vi "適應性控制_輸入權重係數+數位積分_隔振V3(實際控制).vi"() -> ()   [LabVIEW 2010]
uses:
  <vilib>/DAQmx/read.llb/DAQmx Read (Analog DBL 1Chan 1Samp).vi
  <vilib>/DAQmx/write.llb/DAQmx Write (Analog DBL 1Chan 1Samp).vi
  <vilib>/DAQmx/create/channels.llb/DAQmx Create Channel (AI-Voltage-Basic).vi
  <vilib>/DAQmx/configure/timing.llb/DAQmx Timing (Sample Clock).vi
  <vilib>/DAQmx/create/channels.llb/DAQmx Create Channel (AO-Voltage-Basic).vi
  <vilib>/daqmx/miscellaneous.llb/DAQmx Fill In Error Info.vi
  <vilib>/measure/maspectr.llb/FFT Spectrum (Mag-Phase) for 1 Chan.vi
  <vilib>/measure/NI_MAPro.lvlib
panel:
  out "當下頻率":dbl
  out "max value":dbl
  out "phase":cluster{"f0":dbl, "df":dbl, "phase":dbl[]} {"phase" format="%.2p"; "f0" format="%0.2p"; "df" format="%0.2p"}
  in  "averaging parameters 2":T1={"averaging mode"=enum."No averaging", "weighting mode"=enum."Exponential", "number of averages"=10} {"number of averages" min=1}
  out "Waveform Graph 2":cluster{"f0":dbl, "df":dbl, "magnitude":dbl[]}(graph)
  in  "資料數":i32
  in  "權重":dbl[][](array[numeric])=array3077x82[252314 elements]
  in  "輸出DC濾除":dbl
  out "當前權重":dbl[](array[numeric])
  in  "相位":dbl
  in  "I增益":dbl
  in  "DAQ input":tag
  in  "DAQ output":tag
  in  "平均數":i32=1
  in  "ÂoDC«á©ñ¤j":dbl=1.0
  in  "Kp":dbl
  out "當下誤差":dbl=0.1 format="%#_13g"
  out "模擬輸入x(t)":dbl[][](graph)
  out "理想與FIR輸出":dbl[][](graph)
  out "message":string=" INSTRUCTIONS:\r\rNormal Use:  When using subVIs that incorporate the error in/error out (or error I/O) structure, place this handler where you want to inform the user of an error, typically at the end of the I/O data path, as the last action of the program.  If the error in error? is ERROR, the handler creates a message describing the error and its source.  If the type of dialog = 1 (default), the message is displayed to the user, who can only acknowedge it.  If the type = 2, the user can acknowledge the message or abort execution; aborting a program with active I/O is not recommended.  If the type = 0, no message is displayed; this is used to process the error programmatically, and the error out cluster elements are wired to individual terminals for that reason.  \r\rOther Use:\n\r\nlocal testing.  To test the error code of a subVI or function that does not have the error I/O structure, you can wire its error code and a source string to the local error code and error source inputs.  If error in error? indicates no error and error code is not equal to 0, the local code and source are substituted for the error in values, and error? is set TRUE (ERROR)."
  out "誤差":dbl(graph)
  out "while平均運行時間":dbl
  out "收斂time":dbl
  out "各頻率誤差已達標準":bool
  in  "各頻率誤差低於多少亮燈":dbl=0.1 format="%#_13g"
  in  "order":i32=80
  in  "取樣頻率":dbl=1000.0 min=1.0 max=1000.0 step=1.0
  in  "stop":bool
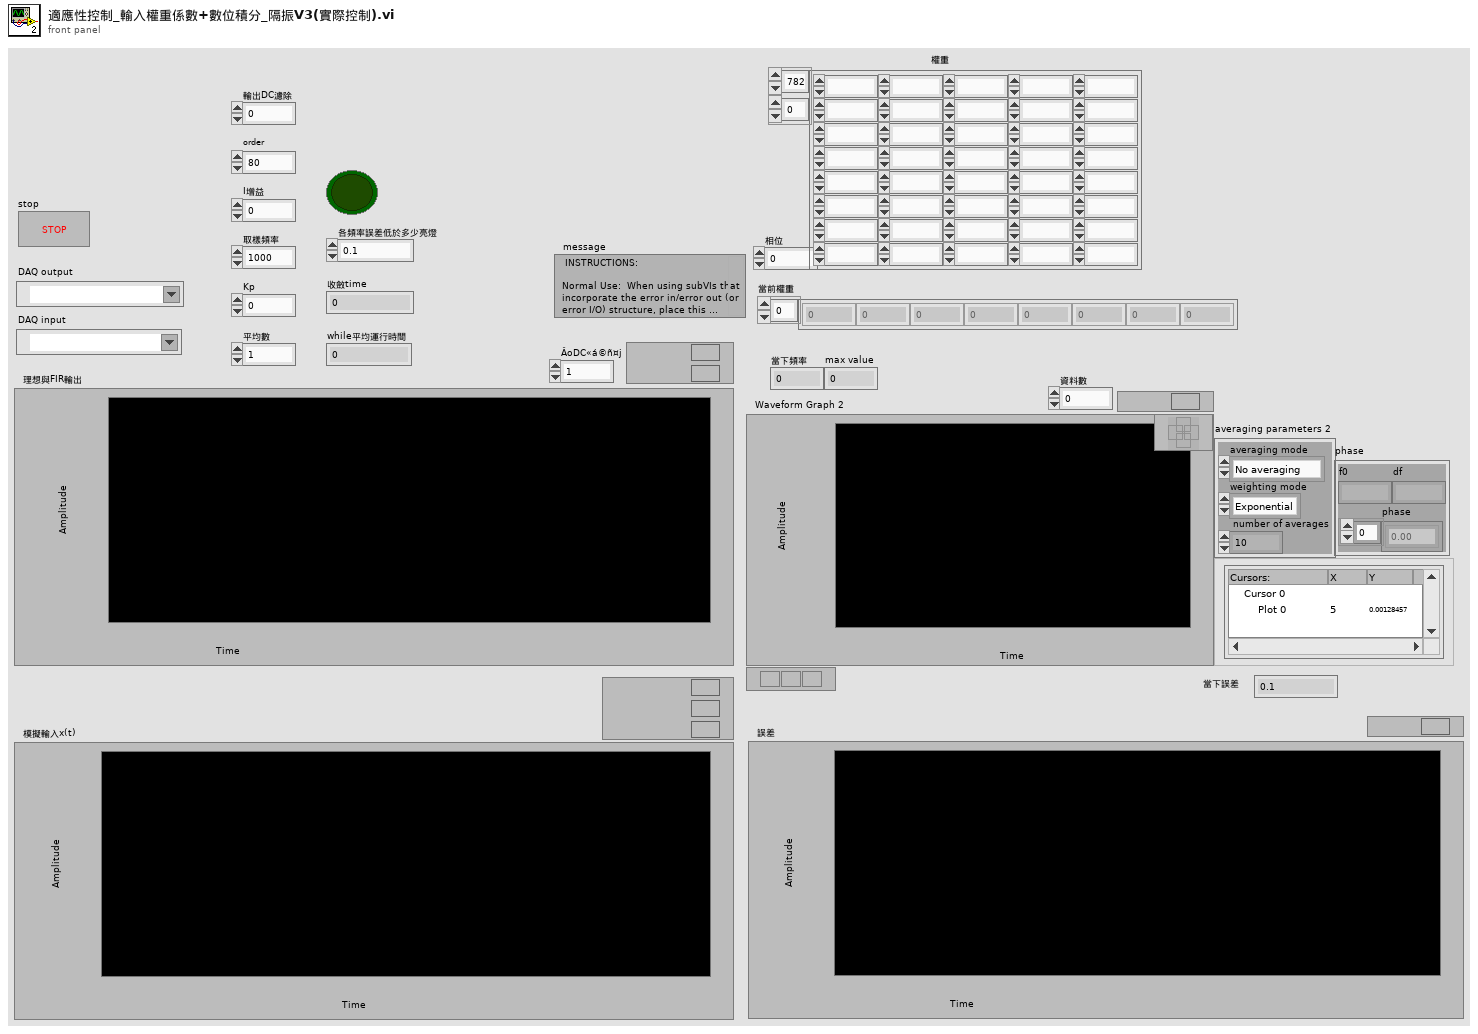
[diagram p1: front panel]
types:
  T1 = cluster{"averaging mode":enum16{"No averaging", "Vector averaging", "RMS averaging", "Peak hold"}, "weighting mode":enum16{"Linear", "Exponential"}, "number of averages":u32}
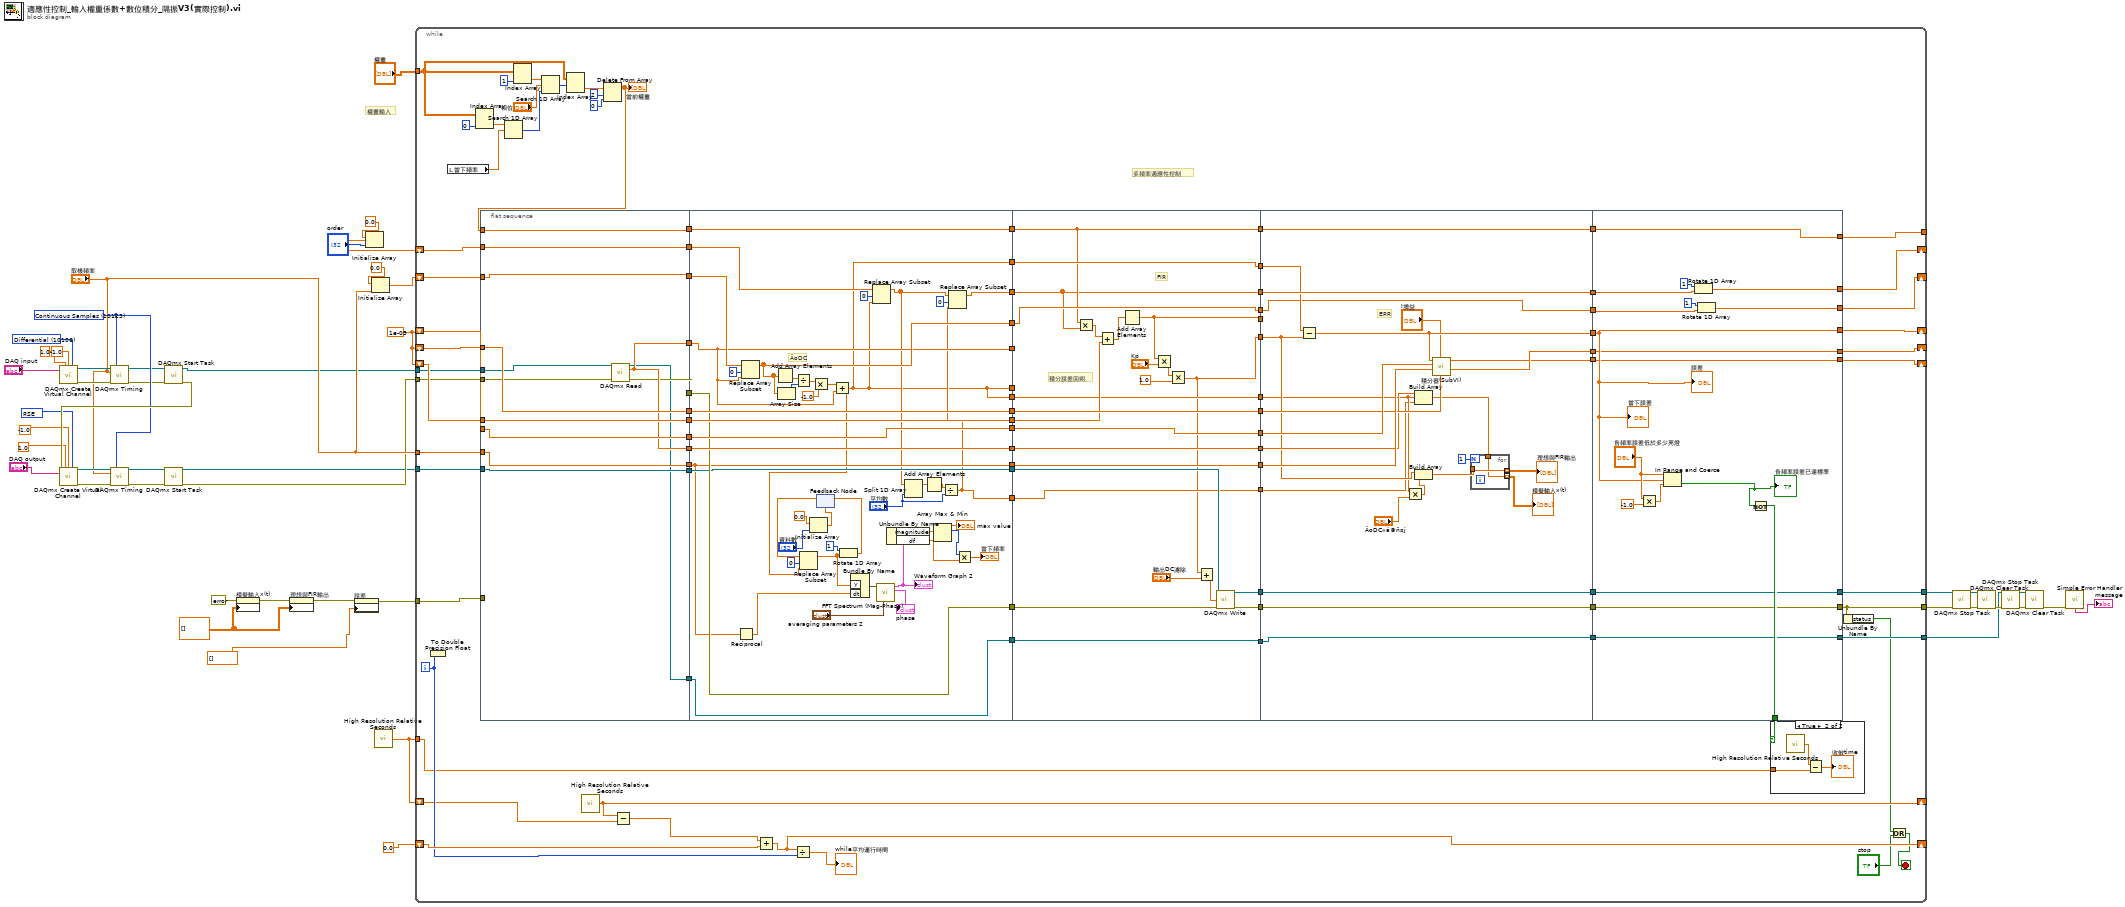
[diagram p0: block diagram]
diagram:
  w29 = 10123 items=["Finite Samples"=10178, "Continuous Samples"=10123, "Hardware Timed Single Point"=12522] ("sample mode")
  w26 = 10083 items=["Default"=-1, "RSE"=10083, "Differential"=10106, "Pseudodifferential"=12529] ("output terminal configuration")
  w25 = 10106 items=["default"=-1, "RSE"=10083, "NRSE"=10078, "Differential"=10106, "Pseudodifferential"=12529] ("input terminal configuration")
  w37 = 1e-05 ("x")
  w33 = dbl[][] [] ("History Data")
  # "權重輸入"
  n1 = call-poly <vilib>:"DAQmx Create Virtual Channel.vi"("maximum value"=1.0, "minimum value"=-1.0, "input terminal configuration"=w25, "physical channels"="DAQ input") -> ("task out"=w17:refnum<k21>, "error out"=w20:errorcluster)  [unwired: 10 in]
  n2 = call-poly <vilib>:"DAQmx Timing.vi"("task/channels in"=w17, "sample mode"=w29, "rate"="取樣頻率", "error in"=w20) -> ("task out"=w18:refnum<k21>, "error out"=w19:errorcluster)  [unwired: 10 in]
  n3 = call <vilib>:"DAQmx Start Task.vi"("task/channels in"=w18, "error in"=w19) -> ("task out"=w15:refnum<k21>, "error out"=w32:errorcluster)  [unwired: 12 in]
  n4 = call-poly <vilib>:"DAQmx Create Virtual Channel.vi"("maximum value"=1.0, "minimum value"=-1.0, "output terminal configuration"=w26, "physical channels"="DAQ output", "error in"=w32) -> ("task out"=w24:refnum<k21>, "error out"=w21:errorcluster)  [unwired: 9 in]
  n5 = call-poly <vilib>:"DAQmx Timing.vi"("task/channels in"=w24, "sample mode"=w29, "rate"="取樣頻率", "error in"=w21) -> ("task out"=w23:refnum<k21>, "error out"=w22:errorcluster)  [unwired: 10 in]
  n6 = call <vilib>:"DAQmx Start Task.vi"("task/channels in"=w23, "error in"=w22) -> ("task out"=w13:refnum<k21>, "error out"=w14:errorcluster)  [unwired: 12 in]
  n7 = property on="模擬輸入x(t)" class="WFChart (strict)"(error in=errorcluster {"status"=FALSE, "code"=0, "source"=""} ("error constant"), "History Data"=w33) -> (error out=w41:errorcluster)  [unwired: 1 in, 1 out]
  n8 = property on="理想與FIR輸出" class="WFChart (strict)"(error in=w41, "History Data"=w33) -> (error out=w42:errorcluster)  [unwired: 1 in, 1 out]
  n9 = property on="誤差" class="WFChart (strict)"(error in=w42, "History Data"=dbl[] []) -> (error out=w44:errorcluster)  [unwired: 1 in, 1 out]
  n10 = Initialize Array(0.0 ("element"), "order") -> (w36:dbl[])
  n11 = Initialize Array(0.0 ("element"), "取樣頻率") -> (w34:dbl[])
  n12 = call <vilib>:"High Resolution Relative Seconds.vi"() -> ("relative seconds"=w46:dbl)
  n13 = while {
    shift-right: [w118] -> _
    shift-left: w36 -> [w142]
    tunnel: w46 -> [w126]
    shift-right: [w127] -> _
    shift-left: w46 -> [w125]
    shift-right: [w128] -> _
    shift-left: 0.0 -> [w130]
    tunnel: w44 -> [w122]
    shift-right: [w116] -> _
    shift-left: w37 -> [w112]
    shift-right: [w108] -> _
    shift-left: w37 -> [w103]
    shift-right: [w102] -> _
    shift-left: w37 -> [w98]
    tunnel: "取樣頻率" -> [w97]
    tunnel: [w92] -> _
    shift-right: [w89] -> _
    shift-left: w34 -> [w91]
    tunnel: w15 -> [w81]
    tunnel: w14 -> [w80]
    tunnel: w13 -> [w79]
    tunnel: [w74] -> w7
    tunnel: [w64] -> w6
    tunnel: [w67] -> w5
    tunnel: "權重" -> [w50]
    i -> [w129]
    stop <- w66 stop-if-true
    # "多頻率適應性控制"
    n14 = To Double Precision Float(number=w129) -> ()  [unwired: 1 out]
    n15 = local read "當下頻率"() -> (w48:dbl)
    n16 = Index Array(array=w50, index (col)=0 ("disabled index (col)")) -> (element=w59:dbl[])  [unwired: 1 in]
    n17 = flat-sequence {
      tunnel: [w159] -> w143
      tunnel: w142 -> [w159]
      tunnel: [w150] -> w141
      tunnel: [w158] -> w138
      tunnel: w49 -> [w158]
      tunnel: w122 -> [_]
      tunnel: [w150] -> w119
      tunnel: [w157] -> w113
      tunnel: w112 -> [w157]
      tunnel: [w156] -> w109
      tunnel: w97 -> [w156]
      tunnel: [w155] -> w104
      tunnel: w103 -> [w155]
      tunnel: [w154] -> w99
      tunnel: w98 -> [w154]
      tunnel: [w149] -> w96
      tunnel: w91 -> [w153]
      tunnel: [w153] -> w90
      tunnel: w81 -> [w152]
      tunnel: w80 -> [w151]
      tunnel: w79 -> [w148]
      tunnel: [w148] -> w77
      tunnel: [w147] -> w70
      tunnel: w143 -> [w204]
      tunnel: w141 -> [w184]
      tunnel: [w182] -> w140
      tunnel: [w205] -> w139
      tunnel: w138 -> [w205]
      tunnel: [w198] -> w123
      tunnel: [w203] -> w120
      tunnel: w119 -> [w203]
      tunnel: [w201] -> w114
      tunnel: w113 -> [w201]
      tunnel: [w185] -> w110
      tunnel: w109 -> [w185]
      tunnel: [w200] -> w105
      tunnel: w104 -> [w200]
      tunnel: [w199] -> w100
      tunnel: w99 -> [w199]
      tunnel: w96 -> [w198]
      tunnel: [w172] -> w94
      tunnel: w90 -> [w196]
      tunnel: [w186] -> w86
      tunnel: [w172] -> w85
      tunnel: [w172] -> w83
      tunnel: [w180] -> w82
      tunnel: [w187] -> w78
      tunnel: w77 -> [w187]
      tunnel: [w171] -> w71
      tunnel: w70 -> [w171]
      tunnel: [w184] -> w61
      tunnel: w140 -> [w210]
      tunnel: w139 -> [w212]
      tunnel: [w212] -> w137
      tunnel: [w211] -> w136
      tunnel: [w210] -> w135
      tunnel: w123 -> [w217]
      tunnel: [w209] -> w121
      tunnel: w120 -> [w209]
      tunnel: [w230] -> w115
      tunnel: w114 -> [w230]
      tunnel: [w229] -> w111
      tunnel: w110 -> [w229]
      tunnel: [w228] -> w106
      tunnel: w105 -> [w228]
      tunnel: w100 -> [w226]
      tunnel: [w222] -> w95
      tunnel: w94 -> [w222]
      tunnel: [w206] -> w93
      tunnel: [w220] -> w87
      tunnel: w86 -> [w220]
      tunnel: w85 -> [w221]
      tunnel: [w221] -> w84
      tunnel: w83 -> [_]
      tunnel: w82 -> [w213]
      tunnel: w78 -> [w218]
      tunnel: [w216] -> w75
      tunnel: [w215] -> w73
      tunnel: w71 -> [w214]
      tunnel: [w214] -> w69
      tunnel: [w213] -> w62
      tunnel: w61 -> [_]
      tunnel: w137 -> [w250]
      tunnel: w136 -> [_]
      tunnel: w135 -> [w252]
      tunnel: [w252] -> w134
      tunnel: [w248] -> w133
      tunnel: w121 -> [w241]
      tunnel: [w250] -> w117
      tunnel: w115 -> [w249]
      tunnel: w111 -> [w247]
      tunnel: [w246] -> w107
      tunnel: w106 -> [w245]
      tunnel: [w244] -> w101
      tunnel: w95 -> [w243]
      tunnel: w93 -> [w239]
      tunnel: [w242] -> w88
      tunnel: w87 -> [w242]
      tunnel: w84 -> [w238]
      tunnel: [w235] -> w76
      tunnel: w75 -> [w235]
      tunnel: w73 -> [w234]
      tunnel: [w234] -> w72
      tunnel: w69 -> [w233]
      tunnel: [w233] -> w68
      tunnel: w62 -> [w232]
      tunnel: w134 -> [w269]
      tunnel: [w275] -> w118
      tunnel: w133 -> [w266]
      tunnel: [w271] -> w124
      tunnel: [w267] -> w92
      tunnel: w117 -> [w267]
      tunnel: [w266] -> w116
      tunnel: [w265] -> w108
      tunnel: w107 -> [w265]
      tunnel: [w264] -> w102
      tunnel: w101 -> [w264]
      tunnel: [w262] -> w89
      tunnel: w88 -> [w261]
      tunnel: w76 -> [w260]
      tunnel: [w260] -> w74
      tunnel: [w259] -> w64
      tunnel: w72 -> [w259]
      tunnel: w68 -> [w258]
      tunnel: [w258] -> w67
      frame #0 {
        n18 = call-poly <vilib>:"DAQmx Read.vi"("task/channels in"=w152, "error in"=w151) -> ("task out"=w147:refnum<k21>, "data"=w150:dbl, "error out"=w149:errorcluster)  [unwired: 11 in]
      }
      frame #1 {
        # "ÂoDC"
        n19 = Reciprocal(x=w185) -> (1/x=w169:dbl)
        n20 = Replace Array Subset(array=w196, new element=w184, index=0) -> (w186:dbl[])
        n21 = Add Array Elements(numeric array=w186) -> (sum=w195:dbl)
        n22 = Array Size(array=w186) -> (size(s)=w194:i32)
        n23 = Divide(x=w195, y=w194) -> (x/y=w193:dbl)
        n24 = Initialize Array(0.0 ("element"), "資料數") -> (w175:dbl[])
        n25 = Multiply(x=w193, y=-1.0) -> (x*y=w191:dbl)
        n26 = feedback #1(w175) -> (w177:dbl[])
        n27 = Add(x=w191, y=w184) -> (x+y=w172:dbl)
        n28 = Replace Array Subset(array=w177, new element=w172, index=0) -> (w168:dbl[])
        n29 = Rotate 1D Array(1:w168, 2:1 ("n")) -> (0:w178:dbl[])
        n30 = feedback-in #1(w178) -> ()
        n31 = Bundle By Name("Y"=w168, "dt"=w169) -> (w170:waveform(dbl))  [unwired: 1 in]
        n32 = Replace Array Subset(array=w204, new element=w172, index=0) -> (w183:dbl[])
        n33 = call-poly <vilib>:"FFT Spectrum (Mag-Phase).vi"("averaging parameters"="averaging parameters 2", "time signal"=w170) -> ("phase"=→"phase":cluster{"f0":dbl, "df":dbl, "phase":dbl[]}, "magnitude"=w165:cluster{"f0":dbl, "df":dbl, "magnitude":dbl[]})  [unwired: 5 in, 3 out]
        "Waveform Graph 2" <- w165
        n34 = Unbundle By Name(w165) -> ("magnitude"=w164:dbl[], "df"=w161:dbl)
        n35 = Split 1D Array(array=w183, index="平均數") -> (first subarray=w190:dbl[])  [unwired: 1 out]
        n36 = Add Array Elements(numeric array=w190) -> (sum=w189:dbl)
        n37 = Array Max & Min(array=w164) -> (max value=→"max value":dbl, max index (indices)=w162:i32)  [unwired: 2 out]
        n38 = Divide(x=w189, y="平均數") -> (x/y=w180:dbl)
        n39 = Replace Array Subset(array=w183, new element=w180, index=0) -> (w182:dbl[])
        n40 = Multiply(x=w162, y=w161) -> (x*y=→"當下頻率":dbl)
      }
      frame #2 {
        # "積分誤差回朔"
        # "FIR"
        n41 = Multiply(x=w212, y=w210) -> (x*y=w227:dbl[])
        n42 = Add(x=w227, y=w226) -> (x+y=w225:dbl[])
        n43 = Add Array Elements(numeric array=w225) -> (sum=w211:dbl)
        n44 = Multiply(x=w211, y="Kp") -> (x*y=w223:dbl)
        n45 = Multiply(x=w223, y=1.0) -> (x*y=w206:dbl)
        n46 = Add(x=w206, y="輸出DC濾除") -> (x+y=w208:dbl)
        n47 = call-poly <vilib>:"DAQmx Write.vi"("task/channels in"=w218, "data"=w208, "error in"=w217) -> ("task out"=w216:refnum<k21>, "error out"=w215:errorcluster)  [unwired: 10 in, 1 out]
      }
      frame #3 {
        # "ERR"
        n48 = Subtract(x=w243, y=w239) -> (x-y=w248:dbl)
        n49 = Multiply(x=w238, y="ÂoDC«á©ñ¤j") -> (x*y=w236:dbl)
        n50 = Build Array(w241, w238, w232) -> (w240:dbl[])
        n51 = Build Array(w239, w236) -> (w254:dbl[])
        n52 = call "積分器(SubVI).vi"("輸入累加ERR回朔"=w245, "I增益"="I增益", "samples (Hz)"=w247, "前一個ERR"=w249, "當下ERR"=w248) -> ("輸出累加ERR回朔"=w246:dbl, "積分修正量"=w244:dbl)  [unwired: 5 in]
        n53 = for {
          N: 1 -> [_]
          tunnel: [w257] -> w251 mode=indexing
          tunnel: w254 -> [w257]
          tunnel: [w256] -> w253 mode=indexing
          tunnel: w240 -> [w256]
        }
        "理想與FIR輸出" <- w251
        "模擬輸入x(t)" <- w253
      }
      frame #4 {
        n54 = Multiply(x="各頻率誤差低於多少亮燈", y=-1.0) -> (x*y=w272:dbl)
        n55 = In Range and Coerce(upper limit="各頻率誤差低於多少亮燈", x=w266, lower limit=w272) -> (In Range?=w268:bool)  [unwired: 1 out]
        "各頻率誤差已達標準" <- w268
        n56 = Rotate 1D Array(1:w269, 2:1 ("n")) -> (0:w275:dbl[])
        n57 = Rotate 1D Array(1:w261, 2:1 ("n")) -> (0:w262:dbl[])
        n58 = Not(x=w268) -> (.not. x?=w271:bool)
        "誤差" <- w266
        "當下誤差" <- w266
      }
    }
    n59 = Search 1D Array(1D array=w59, element=w48) -> (index of element=w56:i32)  [unwired: 1 in]
    n60 = Index Array(array=w50, index (col)=1 ("disabled index (col)")) -> (element=w57:dbl[])  [unwired: 1 in]
    n61 = Search 1D Array(1D array=w57, element="相位", start index (0)=w56) -> (index of element=w54:i32)
    n62 = Index Array(array=w50, index (row)=w54) -> (element=w53:dbl[])  [unwired: 1 in]
    n63 = call <vilib>:"High Resolution Relative Seconds.vi"() -> ("relative seconds"=w127:dbl)
    n64 = Delete From Array(array=w53, length=2, index=0) -> (array with subset deleted=w49:dbl[])  [unwired: 1 out]
    "當前權重" <- w49
    n65 = Subtract(x=w127, y=w125) -> (x-y=w132:dbl)
    n66 = Add(x=w132, y=w130) -> (x+y=w128:dbl)
    n67 = Divide(x=w128, y=w129) -> (x/y=→"while平均運行時間":dbl)
    n68 = case shown="True" w124 {
      tunnel: w126 -> [_ w144]
      frame False {
      }
      frame True {
        n69 = call <vilib>:"High Resolution Relative Seconds.vi"() -> ("relative seconds"=w146:dbl)
        n70 = Subtract(x=w146, y=w144) -> (x-y=→"收斂time":dbl)
      }
    }
    n71 = Unbundle By Name(w64) -> ("status"=w63:bool)
    n72 = Or(x=w63, y="stop") -> (x .or. y?=w66:bool)
  }
  n73 = call <vilib>:"DAQmx Stop Task.vi"("task/channels in"=w7, "error in"=w6) -> ("task out"=w8:refnum<k21>, "error out"=w9:errorcluster)  [unwired: 12 in]
  n74 = call <vilib>:"DAQmx Clear Task.vi"("task in"=w8, "error in"=w9) -> ("error out"=w12:errorcluster)  [unwired: 13 in]
  n75 = call <vilib>:"DAQmx Stop Task.vi"("task/channels in"=w5, "error in"=w12) -> ("task out"=w11:refnum<k21>, "error out"=w10:errorcluster)  [unwired: 12 in]
  n76 = call <vilib>:"DAQmx Clear Task.vi"("task in"=w11, "error in"=w10) -> ("error out"=w4:errorcluster)  [unwired: 13 in]
  n77 = call <vilib>:"Simple Error Handler.vi"("error in (no error)"=w4) -> ("message"=→"message":string)  [unwired: 4 in, 4 out]
